vi "CVT Enum StaticRead.vi"(3 "error in (no error)":errorcluster, 5 "Tag Name":string) -> (0 "error out":errorcluster, 1 "Value":i32)   [LabVIEW 2010]
uses:
  _SubVIs/TypeDefs/cvt_MemBlock Methods.ctl
  _SubVIs/TypeDefs/cvt_TagList Methods.ctl
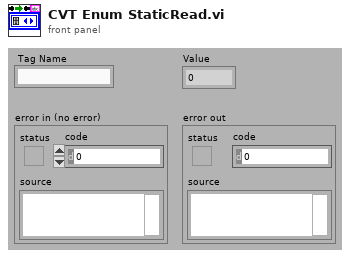
[diagram p1: front panel]
types:
  T1 = typedef "cvt_MemBlock Methods.ctl" = enum16{"init", "read", "readall", "write"}
  T2 = typedef "cvt_TagList Methods.ctl" = enum16{"init", "getindex", "getdesc", "getlist"}
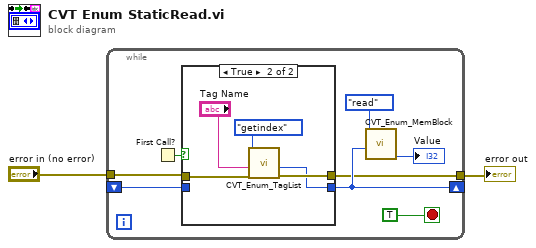
[diagram p0: block diagram]
diagram:
  n1 = while {
    shift-right: [w6] -> _
    shift-left: _ -> [w8]
    tunnel: [w3] -> w2
    tunnel: "error in (no error)" -> [w7]
    stop <- TRUE stop-if-true
    n2 = First Call?() -> (First Call?: T/F=w9:bool)
    n3 = case shown="True" w9 {
      tunnel: [w12 w14] -> w6
      tunnel: w8 -> [w12 _]
      tunnel: w7 -> [w11 w16]
      tunnel: [w11 w15] -> w3
      frame False {
      }
      frame True {
        n4 = call "CVT_Enum_TagList.vi"("error in (no error)"=w16, "Tag Name"="Tag Name", "Method"=cvt_TagList_Methods."getindex") -> ("error out"=w15:errorcluster, "Index"=w14:i32)  [unwired: 1 in, 6 out]
      }
    }
    n5 = call "CVT_Enum_MemBlock.vi"("Index"=w6, "Method"=cvt_MemBlock_Methods."read") -> ("Value"=→"Value":i32)  [unwired: 2 in, 7 out]
  }
  "error out" <- w2
